vi "FPS Calculator.vi"(11 "Average Count":i32=30) -> (3 "fps":dbl)   [LabVIEW 2016]
doc: "Measure the time between calls and average the last few to smooth the value a bit."
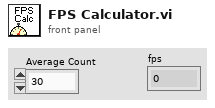
[diagram p1: front panel]
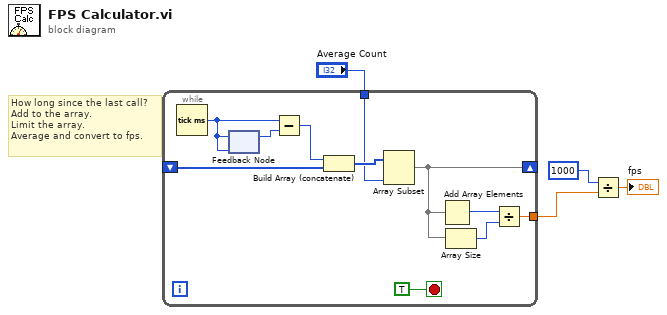
[diagram p0: block diagram]
diagram:
  # "How long since the last call?\nAdd to the array.\nLimit the array.\nAverage and convert to fps."
  n1 = while {
    tunnel: [w12] -> w3
    shift-right: [w5] -> _
    shift-left: _ -> [w11]
    tunnel: "Average Count" -> [w9]
    stop <- TRUE stop-if-true
    n2 = Tick Count (ms)() -> (millisecond timer value=w13:u32)
    n3 = feedback #1(w13) -> (w15:u32)
    n4 = feedback-in #1(w13) -> ()
    n5 = Subtract(x=w13, y=w15) -> (x-y=w6:u32)
    n6 = Build Array (concatenate)(w6, w11) -> (w10:u32[])
    n7 = Array Subset(array=w10, length=w9) -> (w5:u32[])  [unwired: 1 in]
    n8 = Add Array Elements(numeric array=w5) -> (sum=w7:u32)
    n9 = Array Size(array=w5) -> (size(s)=w8:i32)
    n10 = Divide(x=w7, y=w8) -> (x/y=w12:dbl)
  }
  n11 = Divide(x=1000, y=w3) -> (x/y=→"fps":dbl)
